vi "z offset calculation.vi"(11 "z offset in":T1) -> (3 "z offset out":T1)   [LabVIEW 2016]
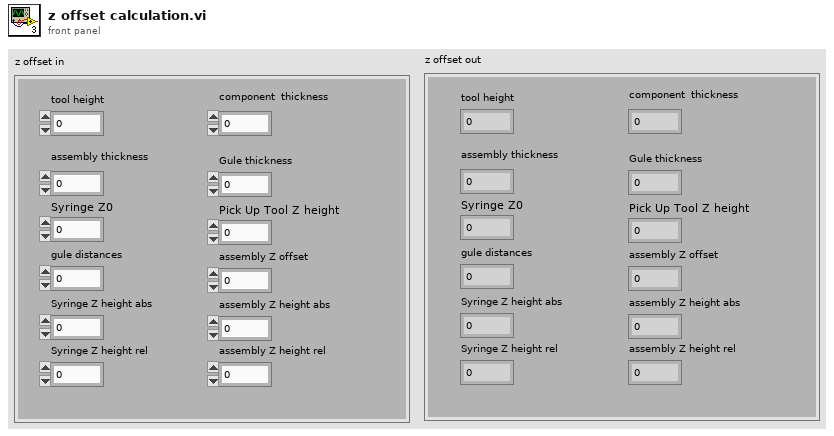
[diagram p1: front panel]
types:
  T1 = cluster{"Syringe Z0":dbl, "assembly thickness":dbl, "tool height":dbl, "Gule thickness ":dbl, "Pick Up Tool Z height":dbl, "assembly Z offset":dbl, "gule distances":dbl, "Syringe Z height abs":dbl, "assembly Z height abs":dbl, "Syringe Z height rel":dbl, "assembly Z height rel":dbl, "component  thickness":dbl}
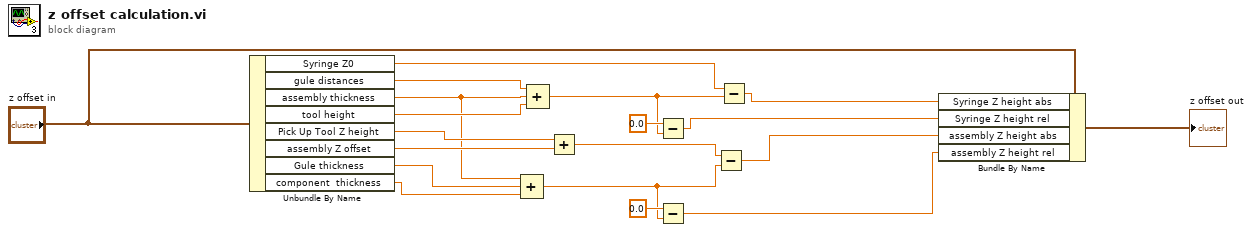
[diagram p0: block diagram]
diagram:
  n1 = Unbundle By Name("z offset in") -> ("Syringe Z0"=w19:dbl, "gule distances"=w8:dbl, "assembly thickness"=w9:dbl, "tool height"=w17:dbl, "Pick Up Tool Z height"=w12:dbl, "assembly Z offset"=w11:dbl, "Gule thickness"=w4:dbl, "component  thickness"=w5:dbl)
  n2 = Compound Arithmetic op=ADD(w9, w4, w5) -> (w2:dbl)
  n3 = Compound Arithmetic op=ADD(w8, w9, w17) -> (w15:dbl)
  n4 = Add(x=w12, y=w11) -> (x+y=w10:dbl)
  n5 = Subtract(x=0.0, y=w15) -> (x-y=w14:dbl)
  n6 = Subtract(x=0.0, y=w2) -> (x-y=w1:dbl)
  n7 = Subtract(x=w10, y=w2) -> (x-y=w13:dbl)
  n8 = Subtract(x=w19, y=w15) -> (x-y=w18:dbl)
  n9 = Bundle By Name(cluster="z offset in", "Syringe Z height abs"=w18, "Syringe Z height rel"=w14, "assembly Z height abs"=w13, "assembly Z height rel"=w1) -> (→"z offset out":T1)
